vi "3_4_Face_Detection_Inference(FPGA)(File).vi"() -> ()   [LabVIEW 2020]
doc: "This example demonstrates the usage of the \"DeepLTK FPGA Addon\" for deploying a Face Detection model on a PXI-FPGA board, utilizing an input image sourced from a file.\n\nMore Examples: https://github.com/ngenehub/deepltk_fpga_examples"
uses:
  <vilib>/Ngene/DeepLTK FPGA Addon/Toolkit/NNF_Host/Low_Level/NNF_Init/Controls/NNF_FPGA_Target_Info.ctl
  <vilib>/userDefined/High Color/nirio_resource_hc.ctl
  <vilib>/Ngene/DeepLTK FPGA Addon/Toolkit/NNF_Host/API/NNF_Set_Input/NNF_Set_Input(2D_U32).vi
  <vilib>/Ngene/DeepLTK FPGA Addon/Toolkit/NNF_Host/Low_Level/NNF_Forward/NNF_Get_CPU_Subnet_Data_from_Variant.vi
  <vilib>/Ngene/DeepLTK FPGA Addon/Toolkit/NNF_Host/Low_Level/NNF_Set_Input/NNF_Copy_Data_to_Buffer(U64).vi
  <vilib>/Ngene/DeepLTK FPGA Addon/Toolkit/NNF_Host/Low_Level/NNF_Set_Input/NNF_Copy_Data_to_Buffer(U32).vi
  <vilib>/FPGAPlugInAG/Dynamic/niLvFpga_Download_Dynamic.vi
  <vilib>/FPGAPlugInAG/Dynamic/niLvFpga_Run_Dynamic.vi
  <vilib>/Ngene/Deep Learning Toolkit/Toolkit/NN_Network/API/NN_Set_Input.vi
  <vilib>/Ngene/Deep Learning Toolkit/Toolkit/NN_Network/API/NN_Set_Input/3D/NN_Set_Input(3D_SGL_idx).vi
  <vilib>/Ngene/DeepLTK FPGA Addon/Toolkit/NNF_Host/Low_Level/NNF_Common/SubVIs/NNF_GLobal.vi
  <vilib>/FPGAPlugInAG/Dynamic/niLvFpga_Close_Dynamic.vi
  <vilib>/rvi/interface/nirviMethod/nirviMethod.xnode
  <vilib>/rvi/interface/nirviCloseFPGA/nirviCloseFPGA.xnode
  <vilib>/vision/NI_Vision_Development_Module.lvlib
  <vilib>/Ngene/Deep Learning Toolkit/Toolkit/Deep_Learning_Toolkit_by_Ngene.lvlib
  <vilib>/Ngene/DeepLTK FPGA Addon/Toolkit/DeepLTK_FPGA_Addon.lvlib
  <vilib>/ptbypt/NI_PtbyPt.lvlib
panel:
  in  "FPGA Bitfile":path=path "D:/Ngene/GitHub/deepltk_fpga_examples/FPGA Bitfiles/NNF_sbRIO_9609_8Cores.lvbitx"
  in  "FPGA Target":T1="rio://10.0.0.39/RIO0" caption="RIO Device"
  out "Loop time":dbl=0.08325622190000104 format="%#_4p"
  out "Target Information":T2={"BRAM _Buff_1_Size"=52500, "BRAM _Buff_2_Size"=45937, "Version"=[8, 1, 1, 0], "# Cores"=8}
  out "Display":T3(plugin-control)
  in  "Scalers File Path":path=path "D:/Ngene/GitHub/deepltk_fpga_examples/2_Face_Detection(PXI,sbRIO)/Models/Face_Detection_NNF_Converted/NNF_Face_Detection_Scalers.cfg"
  out "Inference time":dbl=0.009569441800022106 format="%#_4p"
  out "Sample Path":path=path "D:/Ngene/GitHub/deepltk_fpga_examples/2_Face_Detection(PXI,sbRIO)/Dataset/Images/39_Ice_Skating_Ice_Skating_39_203.jpg"
  in  "Select Sample":i32 min=0 max=19 step=1
  in  "Dataset Path (Images)":path=path "D:/Ngene/GitHub/deepltk_fpga_examples/2_Face_Detection(PXI,sbRIO)/Dataset/Images"
  in  "Confidence_Thresh":sgl=0.39999998
  in  "IOU_Thresh":sgl=0.3
  in  "Stop":bool
  in  "Model Weights":path=path "D:/Ngene/GitHub/deepltk_fpga_examples/2_Face_Detection(PXI,sbRIO)/Models/Face_Detection_NNF_Converted/NNF_Face_Detection.bin"
  in  "Model Topology (CFG)":path=path "D:/Ngene/GitHub/deepltk_fpga_examples/2_Face_Detection(PXI,sbRIO)/Models/Face_Detection_NNF_Converted/NNF_Face_Detection.cfg"
  # "Overview: \nThis example demonstrates the usage of the \"DeepLTK FPGA Addon\" for deploying a Face Detection model on a PXI-FPGA board, utilizing an input image sourced from a file.\nRequirements: \n• DeepLTK - Deep Learning Toolkit for LabVIEW (https://www.ngene.co/deep-learning-toolkit-for-labview)\n• DeepLTK FPGA Addon (https://www.ngene.co/deepltk-accelerator-for-fpga)\n• NI Vision Development Module\n• NI FPGA Module"
  # "Instructions:\nNote: To run the example on RT target copy converted model  and FPGA bitfile to the RT target. \n1.\tSelect FPGA target at FPGA Target control.\n2.\tProvide path to compiled FPGA bitfile at FPGA Bitfile control.  A sample is available in the \"Examples\\FPGA Bitfiles\" folder. \n3. Provide paths to .cfg, .bin and scalers.cfg files generated during model conversion or sample from project (locted in \"Models\\Face_Detection_NNF_Converted\" folder ) at Network Configuration File Path, Weight File Path and Scalers File Path controls.\n4.\tProvide the path to the folder with test images in the \"Dataset Path (Images)\" control. A sample is available in the \"Dataset\" folder.  \n4.\tRun the VI. \n6.\tChange \"Select Sample\" value to select different image samples from the datset.\n7.\tObserve the detections drawn on the \"Display\". The info on the top left of each bounding box\n8. Hit \"Stop\" button to stop the VI\nMore Examples: https://github.com/ngenehub/deepltk_fpga_examples"
  # "Copy resource path from NI MAX if needed"
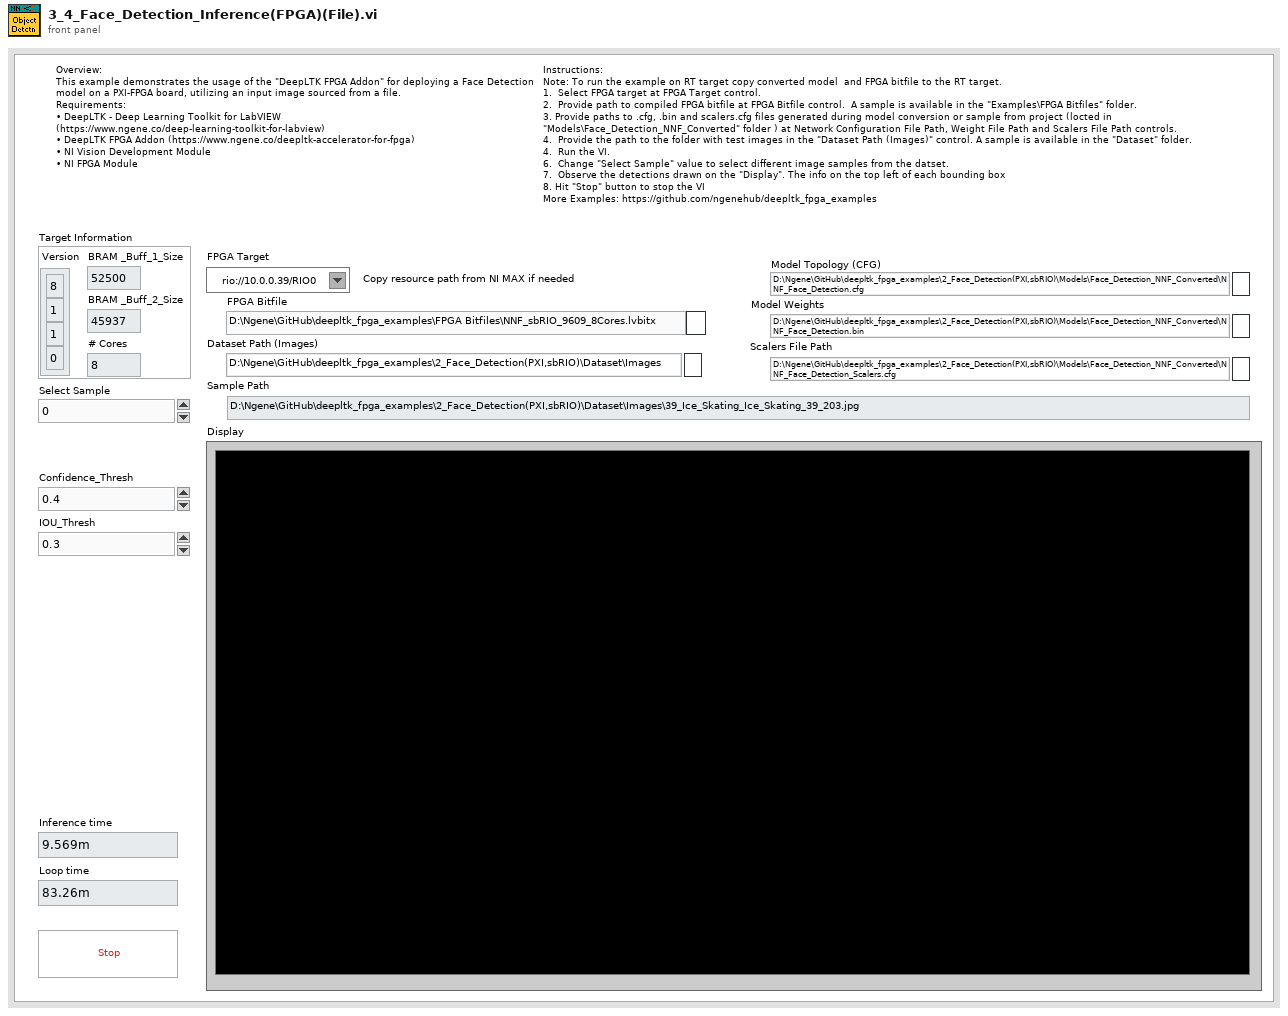
[diagram p1: front panel]
types:
  T1 = typedef "nirio_resource_hc.ctl" = tag
  T2 = typedef "DeepLTK_FPGA_Addon.lvlib/NNF_FPGA_Target_Info.ctl" = cluster{"BRAM _Buff_1_Size":u32, "BRAM _Buff_2_Size":u32, "Version":u8[], "# Cores":u32}
  T3 = typedef "IMAQ Image.ctl" = refnum<image>
  T4 = typedef "Image Type" = u32
  T5 = typedef "DeepLTK_FPGA_Addon.lvlib/NNF.ctl" = cluster{"FPGA VI Ref ":refnum<k20>, "Subnets":T6[], "Dims_In":T8, "#Cores(enum)":T9, "NN_Ref":T10}
  T6 = typedef "DeepLTK_FPGA_Addon.lvlib/NNF_Subnet.ctl" = cluster{"Subnet Type":T7, "Subnet Data":variant, "Input Scaler":sgl, "Output Scaler":sgl}
  T7 = typedef "DeepLTK_FPGA_Addon.lvlib/NNF_Subnet_Type.ctl" = enum16{"CPU", "FPGA", "Split FPGA"}
  T8 = typedef "Deep_Learning_Toolkit_by_Ngene.lvlib/NN_Dims(C,H,W).ctl" = cluster{"C":i32, "H":i32, "W":i32}
  T9 = typedef "DeepLTK_FPGA_Addon.lvlib/NNF_No_Of_Cores.ctl" = enum16{"4CH", "8CH"}
  T10 = typedef "DeepLTK_FPGA_Addon.lvlib/NN_DVR.ctl" = refnum<data-value>
  T11 = typedef "Deep_Learning_Toolkit_by_Ngene.lvlib/NN.ctl" = cluster{"Name":string, "No of Layers":i32, "mBatch":i32, "Layers":T12[], "Dimty":T13, "Dims_In":T8, "Dims_Out":T8, "Working_Dir":path, "Train?":bool, "Train_Params":T14, "LR_Update_Policy":T17, "Session Data":T19, "Ground_truth":T20, "NNg_hdls":T21, "NN_Device":T22, "GPU Id":i32, "Labels":string[], "Receptive Field":T23[], "Loss_Type":T24, "Loss_Cfg_Prms":variant, "NNG_WS":T25}
  T12 = typedef "Deep_Learning_Toolkit_by_Ngene.lvlib/NN_Layer_ref.ctl" = refnum<data-value>
  T13 = typedef "Deep_Learning_Toolkit_by_Ngene.lvlib/NN_In_Out_Dim-ty.ctl" = enum8{"In1D_Out1D", "In3D_Out1D", "In3D_Out3D", "In3D_OutBBox"}
  T14 = typedef "Deep_Learning_Toolkit_by_Ngene.lvlib/NN_Train_Params.ctl" = cluster{"Optimizer":T15, "Beta_1":sgl, "Beta_2":sgl, "Weight Decay(L1)":sgl, "Weight Decay(L2)":sgl, "Data_Sampling":T16}
  T15 = typedef "Deep_Learning_Toolkit_by_Ngene.lvlib/NN_Train_Optimizer.ctl" = enum16{"SGD", "Adam", "Adagrad", "Adadelta", "RMSProp", "Nesterov"}
  T16 = typedef "Deep_Learning_Toolkit_by_Ngene.lvlib/NN_Train_Data_Sampling.ctl" = enum16{"Random", "Sequential"}
  T17 = typedef "Deep_Learning_Toolkit_by_Ngene.lvlib/NN_LR_Policy_Cfg.ctl" = cluster{"Policy_Type":T18, "LR0":dbl, "k":sgl, "WarmUp_Policy":enum16{"Step", "Ramp"}, "WarmUp_Iter":i32, "WarmUp_Ratio":sgl}
  T18 = typedef "Deep_Learning_Toolkit_by_Ngene.lvlib/NN_LR_Policy_Type.ctl" = enum16{"Manual", "Step", "Exp", "1/t"}
  T19 = typedef "Deep_Learning_Toolkit_by_Ngene.lvlib/NN_Train_Session_Data.ctl" = cluster{"Epochs":sgl, "Tot_Iter":i32, "LR":sgl, "LR_iter":i32}
  T20 = typedef "Deep_Learning_Toolkit_by_Ngene.lvlib/NN_Ground_truth.ctl" = cluster{"Y":variant}
  T21 = typedef "Deep_Learning_Toolkit_by_Ngene.lvlib/nng_cuda_handles.ctl" = cluster{"cudnn":u64, "cublas":u64, "stream":u64, "curand":u64}
  T22 = typedef "Deep_Learning_Toolkit_by_Ngene.lvlib/NN_Device.ctl" = enum16{"CPU", "GPU"}
  T23 = typedef "Deep_Learning_Toolkit_by_Ngene.lvlib/NN_Dims(V,H).ctl" = cluster{"V":i32, "H":i32}
  T24 = typedef "Deep_Learning_Toolkit_by_Ngene.lvlib/NN_Loss_Type.ctl" = enum16{"None", "MSE", "CrossEntropy", "YOLO_v2", "YOLO_v4"}
  T25 = typedef "Deep_Learning_Toolkit_by_Ngene.lvlib/NNG_WS.ctl" = cluster{"NNG_WS_Mem":T26, "Max_WS_Size":i64}
  T26 = typedef "Deep_Learning_Toolkit_by_Ngene.lvlib/NNg_WS_Mem_DVR.ctl" = refnum<data-value>
  T27 = typedef "Deep_Learning_Toolkit_by_Ngene.lvlib/NN_Layer.ctl" = cluster{"Name":string, "Layer_Data":variant, "Layer_Type":T28, "Dims_In":T8, "Layers_In":variant, "Dims_Out":T8, "Layers_Out":variant, "Metrics":T29, "GPU_Data":variant, "mBatch":i32, "NN_Device":T22, "NNg_hdls":T21, "Train?":bool, "Dimty":T30, "RecptField":T31}
  T28 = typedef "Deep_Learning_Toolkit_by_Ngene.lvlib/NN_Layer_Type.ctl" = enum16{"Input1D", "Input3D", "Conv1D", "Conv2D", "Conv2D_Adv", "MaxPool", "AvgPool", "UpSample", "DropOut3D", "ShortCut", "Concat", "SoftMax3D", "FC", "DropOut", "Softmax", "Flatten", "YOLO_v2", "YOLO_v4", "Activation", "BatchNormalization", "Unsupported"}
  T29 = typedef "Deep_Learning_Toolkit_by_Ngene.lvlib/NN_Layer_Metrics.ctl" = cluster{"Data":dbl, "Params":dbl, "Ops":dbl}
  T30 = typedef "Deep_Learning_Toolkit_by_Ngene.lvlib/NN_Layer_Dimty.ctl" = enum16{"1D", "3D"}
  T31 = typedef "Deep_Learning_Toolkit_by_Ngene.lvlib/NN_Layer_RF_State.ctl" = cluster{"Dims":T23, "J":T23}
  T32 = typedef "Deep_Learning_Toolkit_by_Ngene.lvlib/NN_BBox_Detection.ctl" = cluster{"Class":i32, "Conf Level":sgl, "BBox":T33}
  T33 = typedef "Deep_Learning_Toolkit_by_Ngene.lvlib/NN_BBox.ctl" = cluster{"x":sgl, "y":sgl, "w":sgl, "h":sgl}
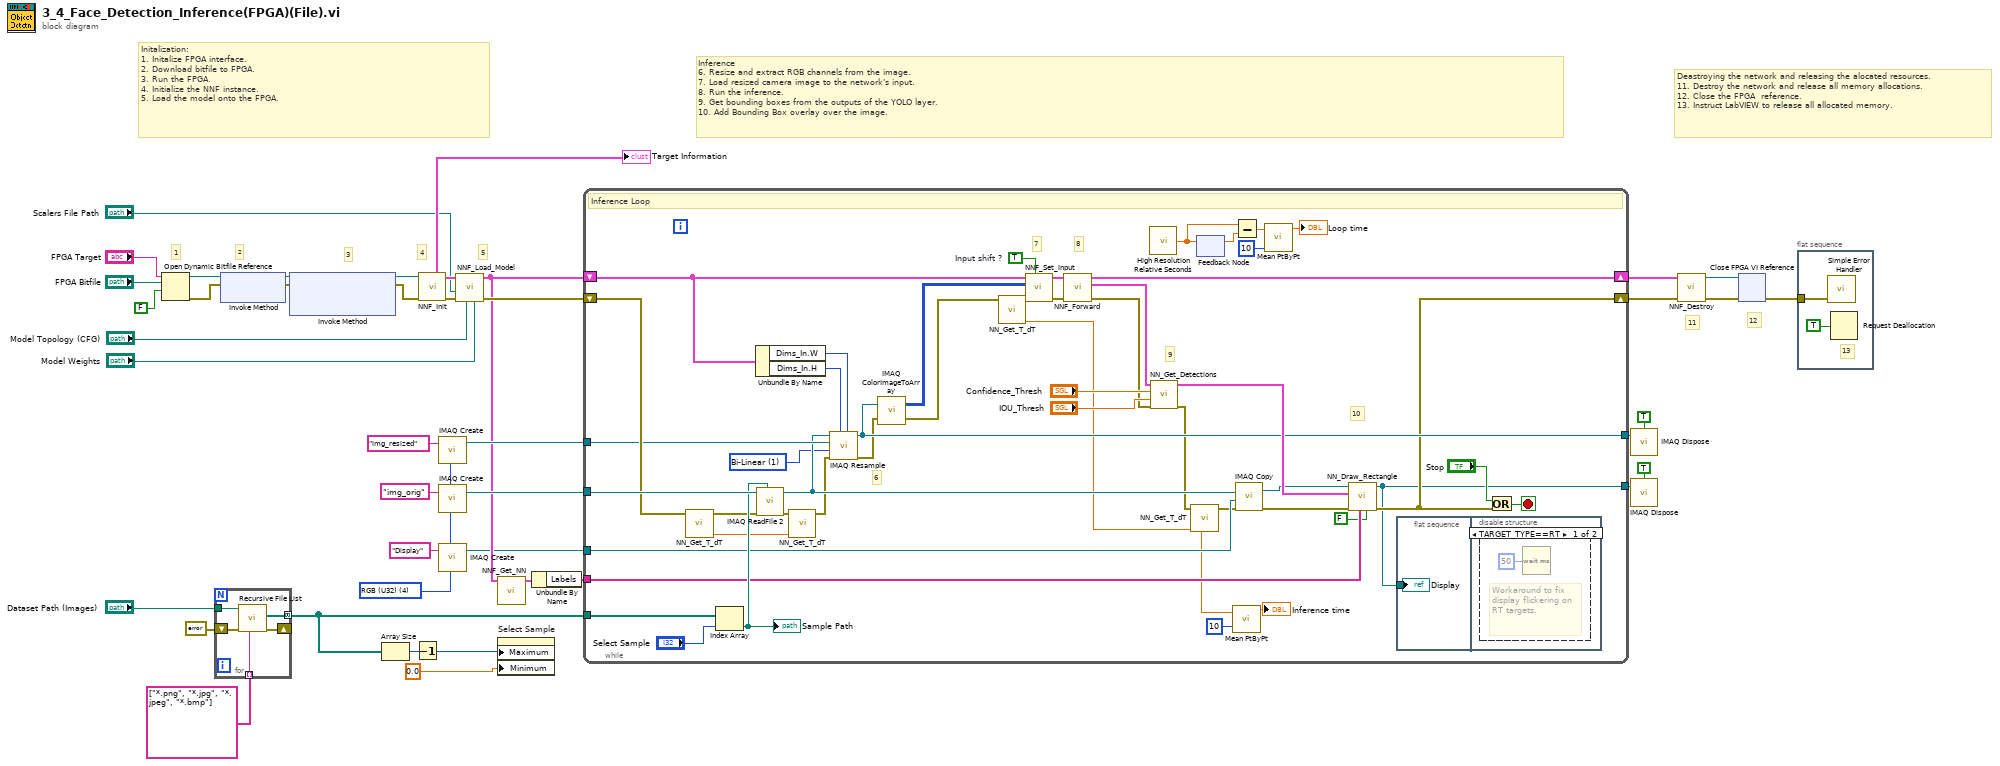
[diagram p0: block diagram]
diagram:
  w2 = T4 4 items=["Grayscale (U8)", "Grayscale (I16)", "Grayscale (SGL)", "Complex (CSG)", "RGB (U32)", "HSL (U32)", "RGB (U64)", "Grayscale (U16)"] ("Image Type")
  # "12"
  # "11"
  # "5"
  # "4"
  # "3"
  # "2"
  # "1"
  # "Deastroying the network and releasing the alocated resources. \n11. Destroy the network and release all memory allocations.\n12. Close the FPGA  reference.\n13. Instruct LabVIEW to release all allocated memory."
  # "Inference\n6.\tResize and extract RGB channels from the image.\n7.\tLoad resized camera image to the network's input.\n8.\tRun the inference.\n9.\tGet bounding boxes from the outputs of the YOLO layer. \n10. Add Bounding Box overlay over the image."
  # "Initalization:\n1. Initalize FPGA interface.\n2. Download bitfile to FPGA.\n3. Run the FPGA.\n4. Initialize the NNF instance.\n5. Load the model onto the FPGA."
  n1 = Open Dynamic Bitfile Reference(0:"FPGA Target", 1:"FPGA Bitfile", 2:FALSE ("Run When Loaded")) -> (5:w25:refnum<k20>, 8:w21:errorcluster)  [unwired: 2 in]
  n2 = for {
    tunnel: "Dataset Path (Images)" -> [w47]
    tunnel: string[] ["*.png", "*.jpg", "*.jpeg", "*.bmp"] ("pattern") -> [w46] mode=indexing
    tunnel: [w45] -> w33 mode=concatenating
    shift-right: [w43] -> _
    shift-left: errorcluster {"status"=FALSE, "code"=0, "source"=""} ("error out") -> [w44]
    n3 = call <vilib>:"Recursive File List.vi"("pattern"=w46, "error in (no error)"=w44, "Folder Path"=w47) -> ("error out"=w43:errorcluster, "All Files in Dir"=w45:path[])  [unwired: 4 in, 3 out]
  }
  n4 = xnode "Invoke Method"("FPGA VI Reference In"=w25, "error in"=w21) -> ("FPGA VI Reference Out"=w22:refnum<k20>, "error out"=w19:errorcluster)
  n5 = xnode "Invoke Method"("FPGA VI Reference In"=w22, "error in"=w19) -> ("FPGA VI Reference Out"=w20:refnum<k20>, "error out"=w18:errorcluster)  [unwired: 1 in]
  n6 = Array Size(array=w33) -> (size(s)=w34:i32)
  n7 = Decrement(x=w34) -> (x-1=w32:i32)
  n8 = call <vilib>:"NNF_Init.vi"("error in"=w18, "FPGA Interface"=w20) -> ("error out"=w26:errorcluster, "NNF out"=w24:T5, "Target Information"=→"Target Information":T2)  [unwired: 7 in]
  n9 = call "IMAQ Create"("Image Name"="img_resized", "Image Type"=w2) -> ("New Image"=w29:T3)  [unwired: 3 in, 1 out]
  n10 = call "IMAQ Create"("Image Name"="img_orig", "Image Type"=w2) -> ("New Image"=w37:T3)  [unwired: 3 in, 1 out]
  n11 = call "IMAQ Create"("Image Name"="Display", "Image Type"=w2) -> ("New Image"=w1:T3)  [unwired: 3 in, 1 out]
  n12 = call <vilib>:"NNF_Load_Model.vi"("Weight File Path"="Model Weights", "Network CFG File Path"="Model Topology (CFG)", "Error in"=w26, "Scalers"="Scalers File Path", "NNF in"=w24) -> ("error Out"=w17:errorcluster, "NNF out"=w5:T5)  [unwired: 5 in]
  n13 = call "NNF_Get_NN.vi"("NNF in"=w5) -> ("NN out"=w4:T11)  [unwired: 10 in]
  n14 = property on="Select Sample" class="DigNum (strict)"("Maximum"=w32, "Minimum"=0.0 ("Data Entry Limits:Minimum")) -> ()  [unwired: 2 in, 2 out]
  n15 = Unbundle By Name(w4) -> ("Labels"=w3:string[])
  n16 = while {
    shift-right: [w82] -> w16
    shift-left: w5 -> [w85]
    tunnel: w33 -> [w92]
    tunnel: w37 -> [w91]
    shift-right: [w50] -> w36
    shift-left: w17 -> [w90]
    tunnel: w29 -> [w84]
    tunnel: [w83] -> w27
    tunnel: w3 -> [w68]
    tunnel: w1 -> [w71]
    tunnel: [w48] -> w41
    stop <- w95 stop-if-true
    w56 = u32 1 items=["Zero Order", "Bi-Linear", "Quadratic", "Cubic Spline"] ("Interpolation Type")
    w78 = TRUE  # Input shift ?
    # "6"
    # "7"
    # "10"
    # "9"
    # "8"
    # "Inference Loop"
    n17 = call <vilib>:"NN_Get_T_dT.vi"("error in (no error)"=w90) -> ("T_out"=w52:dbl, "error out"=w53:errorcluster)  [unwired: 6 in, 1 out]
    n18 = Index Array(array=w92, index="Select Sample") -> (element=w86:path)
    "Sample Path" <- w86
    n19 = Unbundle By Name(w85) -> ("Dims_In.W"=w65:i32, "Dims_In.H"=w64:i32)
    n20 = call "IMAQ ReadFile 2"("File Path"=w86, "error in (no error)"=w53, "Image"=w91) -> ("error out"=w55:errorcluster, "Image Out"=w70:T3)  [unwired: 4 in, 3 out]
    n21 = call <vilib>:"NN_Get_T_dT.vi"("T_in"=w52, "error in (no error)"=w55) -> ("error out"=w54:errorcluster)  [unwired: 5 in, 2 out]
    n22 = call "IMAQ Resample"("X Resolution"=w65, "Y Resolution"=w64, "error in (no error)"=w54, "Interpolation Type"=w56, "Image Dst"=w84, "Image Src"=w70) -> ("error out"=w63:errorcluster, "Image Dst Out"=w83:T3)  [unwired: 4 in]
    n23 = call "IMAQ ColorImageToArray"("Image"=w83, "error in (no error)"=w63) -> ("Image Pixels (U32)"=w79:u32[][], "error out"=w75:errorcluster)  [unwired: 2 in, 1 out]
    n24 = call <vilib>:"NN_Get_T_dT.vi"("error in (no error)"=w75) -> ("T_out"=w49:dbl, "error out"=w74:errorcluster)  [unwired: 6 in, 1 out]
    n25 = call-poly <vilib>:"NNF_Set_Input.vi"("Input shift ?"=w78, "error in"=w74, "Data_in(2D_U32)"=w79, "NNF in"=w85) -> ("error out"=w88:errorcluster, "NNF out"=w89:T5)  [unwired: 6 in]
    n26 = call <vilib>:"NNF_Forward.vi"("error in"=w88, "NNF in"=w89) -> ("error out"=w80:errorcluster, "Last_Layer"=w81:T27, "NNF out"=w82:T5)  [unwired: 7 in]
    n27 = call <vilib>:"High Resolution Relative Seconds.vi"() -> ("relative seconds"=w77:dbl)
    n28 = call <vilib>:"NN_Get_Detections.vi"("error in"=w80, "IOU_Thrsh"="IOU_Thresh", "Confidence_Thrsh"="Confidence_Thresh", "YOLO_Layer"=w81) -> ("error out"=w67:errorcluster, "Detections"=w87:T32[])  [unwired: 6 in]
    n29 = call <vilib>:"NN_Get_T_dT.vi"("T_in"=w49, "error in (no error)"=w67) -> ("error out"=w66:errorcluster, "dT"=w59:dbl)  [unwired: 5 in, 1 out]
    n30 = feedback #1() -> (w76:dbl)  [unwired: 1 in]
    n31 = feedback-in #1(w77) -> ()
    n32 = call <vilib>:"Mean PtByPt.vi"("x"=w59, "sample length"=10) -> ("mean"=→"Inference time":dbl)  [unwired: 2 in, 1 out]
    n33 = Subtract(x=w77, y=w76) -> (x-y=w58:dbl)
    n34 = call "IMAQ Copy"("error in (no error)"=w66, "Image Dst"=w71, "Image Src"=w70) -> ("error out"=w69:errorcluster, "Image Dst Out"=w51:T3)  [unwired: 3 in]
    n35 = call <vilib>:"Mean PtByPt.vi"("x"=w58, "sample length"=10) -> ("mean"=→"Loop time":dbl)  [unwired: 2 in, 1 out]
    n36 = call "NN_Draw_Rectangle.vi"("Clear"=FALSE, "Labels"=w68, "error in (no error)"=w69, "Draw_Boxes"=w87, "Image_in"=w51) -> ("error out"=w50:errorcluster, "Image_out"=w48:T3)  [unwired: 4 in, 1 out]
    n37 = flat-sequence {
      tunnel: w48 -> [w97]
      frame #0 {
        "Display" <- w97
      }
      frame #1 {
        n38 = disable-structure shown="TARGET_TYPE==RT" {
          frame condition #0 {
            # "Workaround to fix display flickering on RT targets."
            n39 = Wait (ms)(milliseconds to wait=u32 50) -> ()  [unwired: 1 out]
          }
          frame condition #1 (active) {
          }
        }
      }
    }
    n40 = Or(x="Stop", y=w50) -> (x .or. y?=w95:bool)
  }
  n41 = call "IMAQ Dispose"("All Images? (No)"=TRUE, "Image"=w27) -> ()  [unwired: 4 in, 1 out]
  n42 = call "IMAQ Dispose"("All Images? (No)"=TRUE, "Image"=w41) -> ()  [unwired: 4 in, 1 out]
  n43 = call <vilib>:"NNF_Destroy.vi"("error in"=w36, "NNF in"=w16) -> ("error out"=w15:errorcluster, "FPGA VI Ref"=w13:refnum<k20>)  [unwired: 8 in]
  n44 = xnode "Close FPGA VI Reference"("FPGA VI Reference In"=w13, "error in"=w15) -> ("error out"=w14:errorcluster)
  n45 = flat-sequence {
    tunnel: w14 -> [w99]
    frame #0 {
      # "13"
      n46 = call <vilib>:"Simple Error Handler.vi"("error in (no error)"=w99) -> ()  [unwired: 4 in, 5 out]
      n47 = Request Deallocation(TRUE ("flag")) -> ()
    }
  }
